vi "Test Call SubVi.vi"() -> ()   [LabVIEW 2024]
panel:
  in  "Numeric":dbl
  out "Gauge":dbl(knob) scale=0.0..10.0
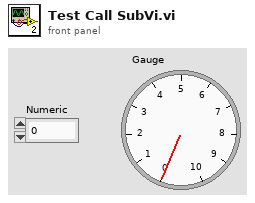
[diagram p1: front panel]
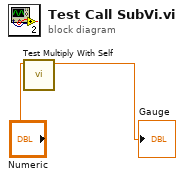
[diagram p0: block diagram]
diagram:
  n1 = call "Test Multiply With Self.vi"("Numeric"="Numeric") -> ("Gauge"=→"Gauge":dbl)  [unwired: 10 in]
